vi "create metadata.vi"(0 "HarpDataFrame":T1, 2 "use system decimal point (T)":bool, 13 "Enum":enum16{"Find Match", "Reset"}(ring)) -> (8 "Line":string, 15 "Metadata Complete":bool)   [LabVIEW 2010]
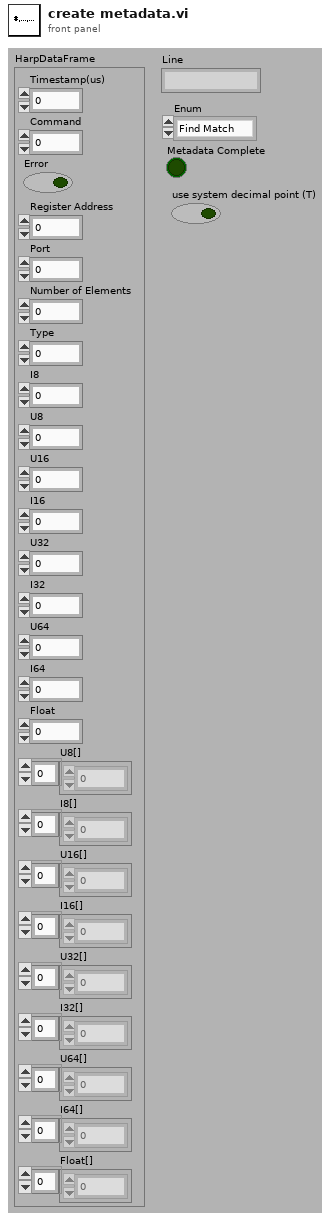
[diagram p1: front panel]
types:
  T1 = cluster{"Timestamp(us)":dbl, "Command":u8, "Error":bool, "Register Address":u8, "Port":u8, "Number of Elements":u8, "Type":u8, "I8":i8, "U8":u8, "U16":u16, "I16":i16, "U32":u32, "I32":i32, "U64":u64, "I64":i64, "Float":sgl, "U8[]":u8[], "I8[]":i8[], "U16[]":u16[], "I16[]":i16[], "U32[]":u32[], "I32[]":i32[], "U64[]":u64[], "I64[]":i64[], "Float[]":sgl[]}
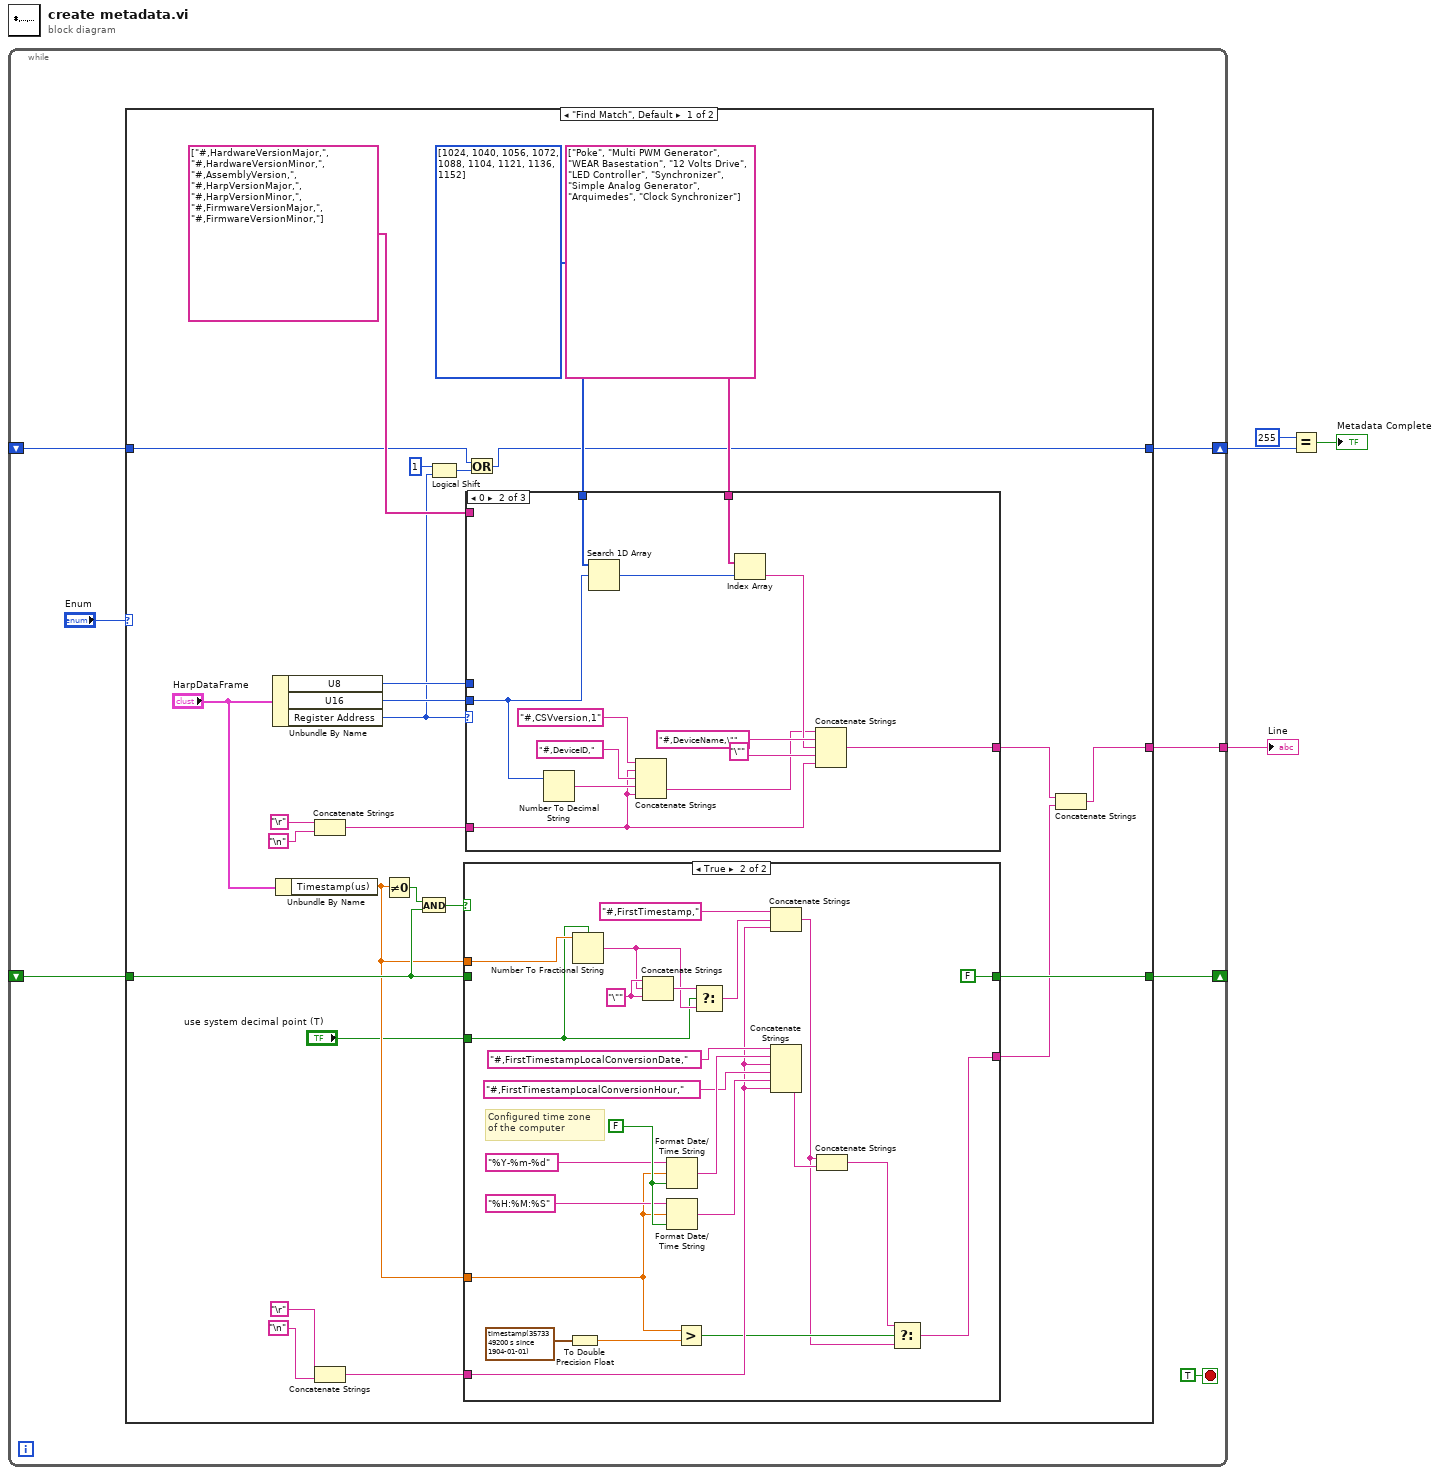
[diagram p0: block diagram]
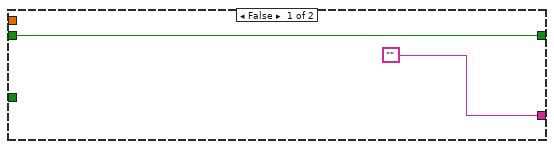
[diagram p2: hidden frame]
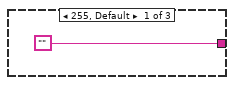
[diagram p3: hidden frame]
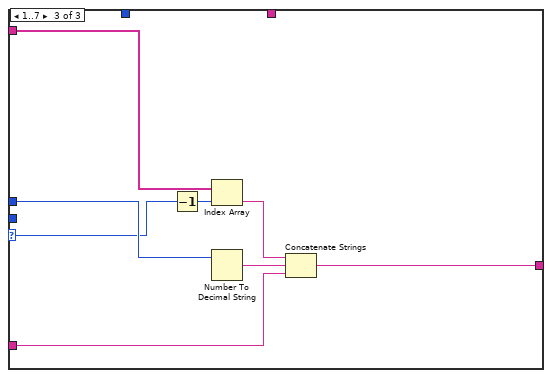
[diagram p4: hidden frame]
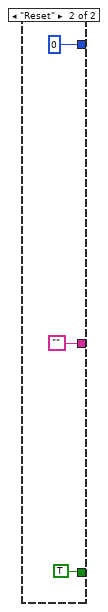
[diagram p5: hidden frame]
diagram:
  n1 = while {
    shift-right: [w9] -> _
    shift-left: _ -> [w7]
    tunnel: [w8] -> w4
    shift-right: [w6] -> w3
    shift-left: _ -> [w5]
    stop <- TRUE ("stop") stop-if-true
    n2 = case shown="\"Find Match\", Default" "Enum" {
      tunnel: [w26 TRUE ("stop")] -> w9
      tunnel: [w21 ""] -> w8
      tunnel: w7 -> [w25 _]
      tunnel: w5 -> [w15 _]
      tunnel: [w13 u8 0 ("U8")] -> w6
      frame "Find Match", Default {
        n3 = Unbundle By Name("HarpDataFrame") -> ("U8"=w36:u8, "U16"=w35:u16, "Register Address"=w16:u8)
        n4 = Unbundle By Name("HarpDataFrame") -> ("Timestamp(us)"=w18:dbl)
        n5 = Concatenate Strings("\r", "\n") -> (w31:string)
        n6 = Concatenate Strings("\r", "\n") -> (w22:string)
        n7 = Not Equal To 0?(x=w18) -> (x != 0?=w28:bool)
        n8 = And(x=w28, y=w25) -> (x .and. y?=w27:bool)
        n9 = Logical Shift(y=i16 1, x=w16) -> (x << y=w14:u8)
        n10 = case shown="True" w27 {
          tunnel: [w39 FALSE ("stop")] -> w26
          tunnel: w25 -> [w39 _]
          tunnel: w18 -> [_ w62]
          tunnel: w22 -> [_ w53]
          tunnel: ["" w46] -> w19
          tunnel: w18 -> [_ w40]
          tunnel: "use system decimal point (T)" -> [_ w41]
          frame False {
          }
          frame True {
            w45 = "\"" ("string")
            w61 = FALSE ("UTC format")
            # "Configured time zone\nof the computer"
            n11 = To Double Precision Float(number=timestamp(3573349200 s since 1904-01-01)) -> (double precision float=w51:dbl)
            n12 = Number To Fractional String(use system decimal point (T)=w41, number=w62) -> (F-format string=w43:string)  [unwired: 2 in]
            n13 = Concatenate Strings(w45, w43, w45) -> (w44:string)
            n14 = Format Date/Time String(time format string (%c)="%Y-%m-%d", seconds (now)=w40, UTC format=w61) -> (date/time string=w58:string)
            n15 = Format Date/Time String(time format string (%c)="%H:%M:%S", seconds (now)=w40, UTC format=w61) -> (date/time string=w55:string)
            n16 = Greater?(x=w40, y=w51) -> (0:w49:bool)
            n17 = Select(t=w44, s=w41, f=w43) -> (s? t:f=w42:string)
            n18 = Concatenate Strings("#,FirstTimestamp," ("string"), w42, w53) -> (w47:string)
            n19 = Concatenate Strings("#,FirstTimestampLocalConversionDate," ("string"), w58, w53, "#,FirstTimestampLocalConversionHour," ("string"), w55, w53) -> (w50:string)
            n20 = Concatenate Strings(w47, w50) -> (w48:string)
            n21 = Select(t=w48, s=w49, f=w47) -> (s? t:f=w46:string)
          }
        }
        n22 = case shown="0" w16 {
          selector: w16 -> [_ _ w78]
          tunnel: u16[] [1024, 1040, 1056, 1072, 1088, 1104, 1121, 1136, 1152] -> [_ w77 _]
          tunnel: w36 -> [_ _ w79]
          tunnel: w35 -> [_ w67 _]
          tunnel: string[] ["Poke", "Multi PWM Generator", "WEAR Basestation", "12 Volts Drive", "LED Controller", "Synchronizer", "Simple Analog Generator", "Arquimedes", "Clock Synchronizer"] -> [_ w76 _]
          tunnel: w31 -> [_ w66 w85]
          tunnel: ["" w71 w80] -> w20
          tunnel: string[] ["#,HardwareVersionMajor,", "#,HardwareVersionMinor,", "#,AssemblyVersion,", "#,HarpVersionMajor,", "#,HarpVersionMinor,", "#,FirmwareVersionMajor,", "#,FirmwareVersionMinor,"] -> [_ _ w82]
          frame 255, Default {
          }
          frame 0 {
            n23 = Number To Decimal String(number=w67) -> (decimal integer string=w70:string)  [unwired: 1 in]
            n24 = Search 1D Array(1D array=w77, element=w67) -> (index of element=w75:i32)  [unwired: 1 in]
            n25 = Concatenate Strings("#,CSVversion,1" ("string"), w66, "#,DeviceID," ("string"), w70, w66) -> (w68:string)
            n26 = Index Array(array=w76, index=w75) -> (element=w73:string)
            n27 = Concatenate Strings(w68, "#,DeviceName,\"" ("string"), w73, "\"" ("string"), w66) -> (w71:string)
          }
          frame 1..7 {
            n28 = Decrement(x=w78) -> (x-1=w83:u8)
            n29 = Index Array(array=w82, index=w83) -> (element=w81:string)
            n30 = Number To Decimal String(number=w79) -> (decimal integer string=w84:string)  [unwired: 1 in]
            n31 = Concatenate Strings(w81, w84, w85) -> (w80:string)
          }
        }
        n32 = Or(x=w15, y=w14) -> (x .or. y?=w13:u8)
        n33 = Concatenate Strings(w20, w19) -> (w21:string)
      }
      frame "Reset" {
      }
    }
  }
  "Line" <- w4
  n34 = Equal?(x=u8 255, y=w3) -> (x = y?=→"Metadata Complete":bool)
